vi "image process.vi"(7 "物理通道":tag="Dev1/ao0", 10 "输出数组":u8[][](array[numeric])) -> ()   [LabVIEW 2014]
uses:
  <vilib>/Utility/error.llb/DialogType.ctl
  <vilib>/DAQmx/create/channels.llb/DAQmx Create Channel (AO-Voltage-Basic).vi
  <vilib>/DAQmx/write.llb/DAQmx Write (Analog DBL 1Chan 1Samp).vi
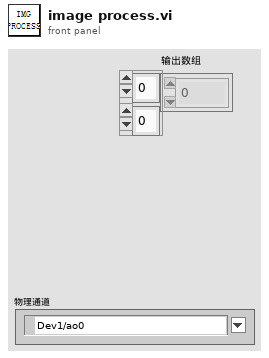
[diagram p1: front panel]
types:
  T1 = typedef "DialogType.ctl" = u16
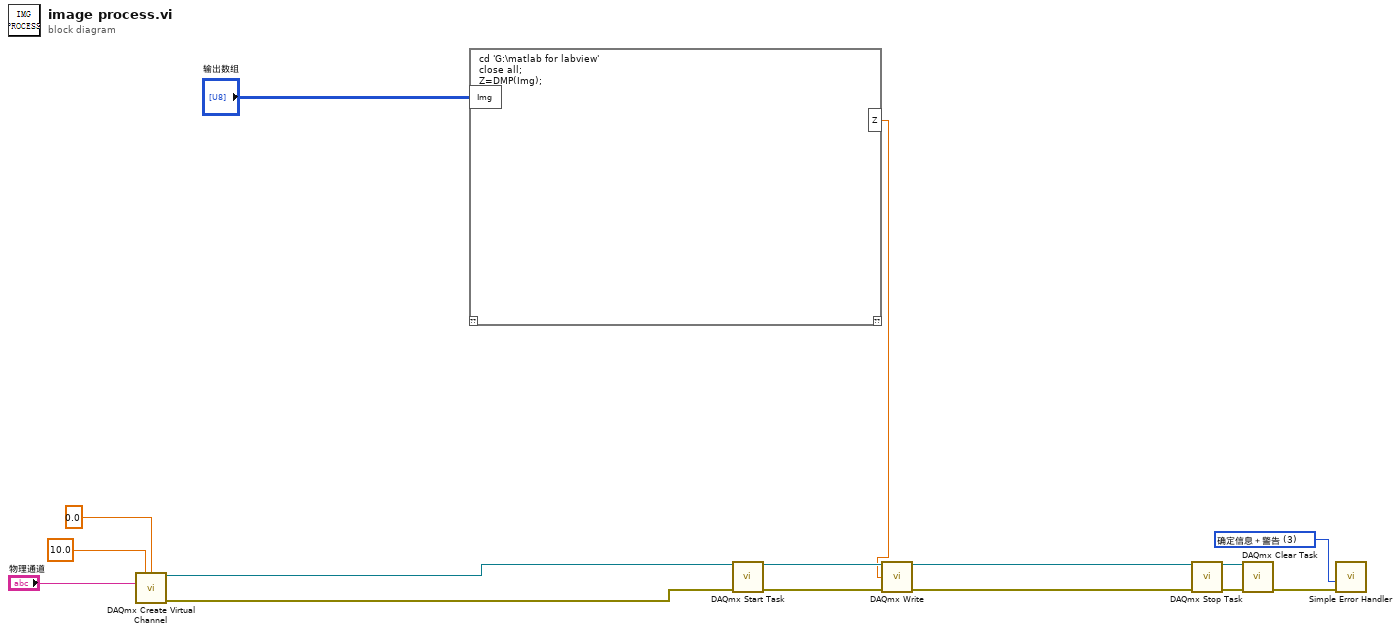
[diagram p0: block diagram]
diagram:
  w4 = T1 3 items=["无对话框", "确定信息", "继续或停止信息", "确定信息＋警告", "继续/停止＋警告"] ("对话框类型（确定信息：1）")
  n1 = call-poly <vilib>:"DAQmx Create Virtual Channel.vi"("maximum value"=10.0 ("最大电压"), "minimum value"=0.0 ("最小电压"), "physical channels"="物理通道") -> ("task out"=w1:refnum<k21>, "error out"=w3:errorcluster)  [unwired: 11 in]
  n2 = script code="cd 'G:\\matlab for labview'\nclose all;\nZ=DMP(Img);"("Img"="输出数组") -> ("Z"=w2:dbl)  [unwired: 1 in, 1 out]
  n3 = call <vilib>:"DAQmx Start Task.vi"("task/channels in"=w1, "error in"=w3) -> ("task out"=w10:refnum<k21>, "error out"=w9:errorcluster)  [unwired: 12 in]
  n4 = call-poly <vilib>:"DAQmx Write.vi"("task/channels in"=w10, "data"=w2, "error in"=w9) -> ("task out"=w8:refnum<k21>, "error out"=w7:errorcluster)  [unwired: 10 in, 1 out]
  n5 = call <vilib>:"DAQmx Stop Task.vi"("task/channels in"=w8, "error in"=w7) -> ("task out"=w6:refnum<k21>, "error out"=w5:errorcluster)  [unwired: 12 in]
  n6 = call <vilib>:"DAQmx Clear Task.vi"("task in"=w6, "error in"=w5) -> ("error out"=w11:errorcluster)  [unwired: 13 in]
  n7 = call <vilib>:"Simple Error Handler.vi"("type of dialog (OK msg:1)"=w4, "error in (no error)"=w11) -> ()  [unwired: 3 in, 5 out]
